vi "HIOKI PW3390 Conf Sync control.vi"(0 "VISA Resource":refnum<visa-resource-name>, 1 "Set/Query (F: Set)":bool, 5 "Control (0: MASTER)":enum16{"MASTER", "SLAVE"}(ring), 7 "Event Type (0: HOLD)":enum16{"HOLD", "SAVE", "COPY"}(ring), 11 "error in (no error)":errorcluster, 12 "OPC query (T: ON)":bool=TRUE, 13 "Error Out (F: Off)":bool) -> (4 "VISA Resource out":refnum<visa-resource-name>, 6 "Control out":enum16{"MASTER", "SLAVE"}(ring), 8 "Event Type out":enum16{"HOLD", "SAVE", "COPY"}(ring), 15 "error out":errorcluster)   [LabVIEW 2009]
doc: "Sets and reads the functions related to the Synchronized Control.\n\nSet/Query\n Set: Send the setting commands for the device.\n Query: Query the setting of the device.\n\nControl\n Sets the Master/Slave of the Synchronized Control.\n\nEvent Type\n Sets the Synchronized Events of the Synchronized Control."
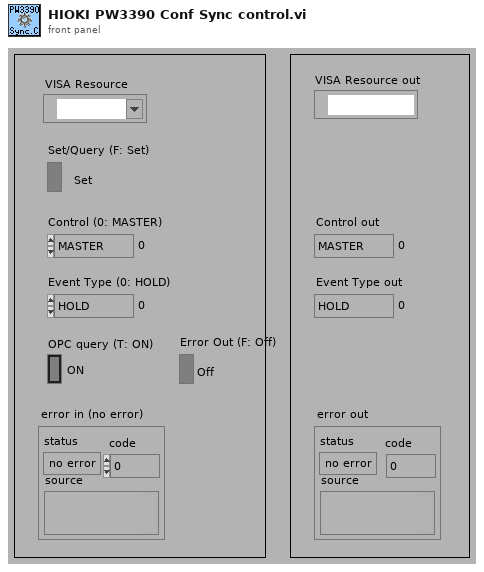
[diagram p1: front panel]
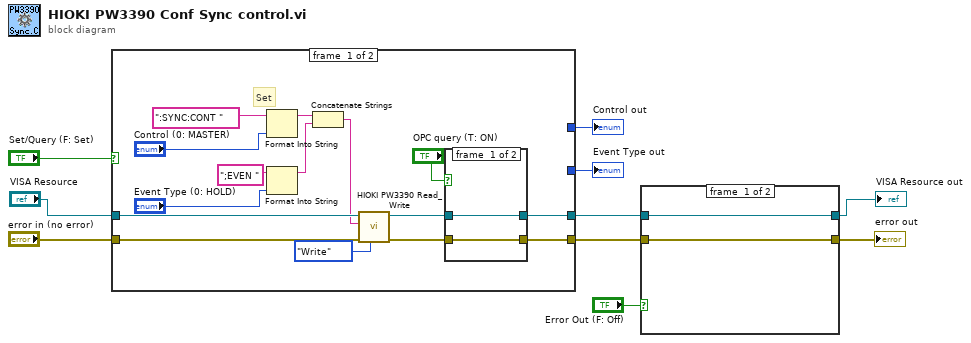
[diagram p0: block diagram]
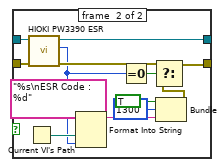
[diagram p2: hidden frame]
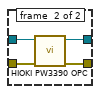
[diagram p3: hidden frame]
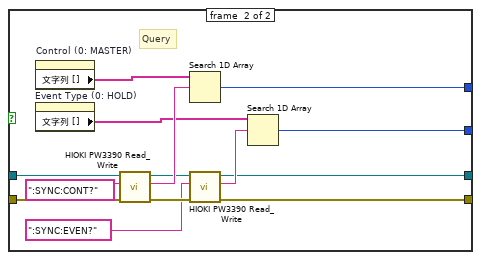
[diagram p4: hidden frame]
diagram:
  n1 = case shown="FALSE" "Set/Query (F: Set)" {
    tunnel: "error in (no error)" -> [w24 w44]
    tunnel: [w11 w37] -> w7
    tunnel: "VISA Resource" -> [w25 w43]
    tunnel: [w12 w36] -> w6
    tunnel: [_ w41] -> w4
    tunnel: [_ w33] -> w3
    frame #0 {
      # "Set"
      n2 = Format Into String(initial string=":SYNC:CONT ", "Control (0: MASTER)") -> (resulting string=w17:string)  [unwired: 2 in, 1 out]
      n3 = Format Into String(initial string=";EVEN ", "Event Type (0: HOLD)") -> (resulting string=w18:string)  [unwired: 2 in, 1 out]
      n4 = Concatenate Strings(w17, w18) -> (w16:string)
      n5 = call <instrlib>:"HIOKI PW3390 Read_Write.vi"("Read/Write"=enum16{"Read", "Write"}."Write", "error in (no error)"=w24, "data in"=w16, "VISA Resource"=w25) -> ("error out"=w13:errorcluster, "VISA Resource out"=w14:refnum<visa-resource-name>)  [unwired: 5 in, 1 out]
      n6 = case shown="TRUE" "OPC query (T: ON)" {
        tunnel: [w27 w31] -> w12
        tunnel: [w26 w30] -> w11
        tunnel: w14 -> [w27 w29]
        tunnel: w13 -> [w26 w28]
        frame #0 {
        }
        frame #1 {
          n7 = call <instrlib>:"HIOKI PW3390 OPC.vi"("error in (no error)"=w28, "VISA Resource"=w29) -> ("error out"=w30:errorcluster, "VISA Resource out"=w31:refnum<visa-resource-name>)  [unwired: 7 in, 1 out]
        }
      }
    }
    frame #1 {
      # "Query"
      n8 = property on="Control (0: MASTER)" class="Enum (strict)"() -> ("文字列 []"=w40:string[])  [unwired: 2 in, 2 out]
      n9 = property on="Event Type (0: HOLD)" class="Enum (strict)"() -> ("文字列 []"=w39:string[])  [unwired: 2 in, 2 out]
      n10 = call <instrlib>:"HIOKI PW3390 Read_Write.vi"("error in (no error)"=w44, "data in"=":SYNC:CONT?", "VISA Resource"=w43) -> ("error out"=w34:errorcluster, "data out"=w42:string, "VISA Resource out"=w35:refnum<visa-resource-name>)  [unwired: 6 in]
      n11 = Search 1D Array(1D array=w40, element=w42) -> (index of element=w41:i32)  [unwired: 1 in]
      n12 = call <instrlib>:"HIOKI PW3390 Read_Write.vi"("error in (no error)"=w34, "data in"=":SYNC:EVEN?", "VISA Resource"=w35) -> ("error out"=w37:errorcluster, "data out"=w38:string, "VISA Resource out"=w36:refnum<visa-resource-name>)  [unwired: 6 in]
      n13 = Search 1D Array(1D array=w39, element=w38) -> (index of element=w33:i32)  [unwired: 1 in]
    }
  }
  "Control out" <- w4
  "Event Type out" <- w3
  n14 = case shown="TRUE" "Error Out (F: Off)" {
    tunnel: w6 -> [w47 w60]
    tunnel: w7 -> [w46 w59]
    tunnel: [w46 w49] -> w5
    tunnel: [w47 w58] -> w1
    frame #0 {
    }
    frame #1 {
      n15 = Current VI's Path() -> (path=w56:path)
      n16 = call <instrlib>:"HIOKI PW3390 ESR.vi"("error in (no error)"=w59, "VISA Resource"=w60) -> ("error out"=w50:errorcluster, "Output Value"=w48:u8, "VISA Resource out"=w58:refnum<visa-resource-name>)  [unwired: 6 in, 1 out]
      n17 = Format Into String(format string="%s\nESR Code : %d", w56, w48) -> (resulting string=w52:string)  [unwired: 2 in, 1 out]
      n18 = Equal To 0?(x=w48) -> (x = 0?=w57:bool)
      n19 = Bundle("status"=TRUE, "code"=1300, w52) -> (w51:cluster{"status":bool, "code":i32, string})  [unwired: 1 in]
      n20 = Select(t=w50, s=w57, f=w51) -> (s? t:f=w49:errorcluster)
    }
  }
  "error out" <- w5
  "VISA Resource out" <- w1
